vi "Execute FTE.vi"(7 "FTE":i64, 8 "error in (no error)":errorcluster, 11 "CIFCorePlugin in":refnum<class "CIFCorePlugin.lvclass">) -> (0 "error out":errorcluster, 3 "CIFCorePlugin out":refnum<class "CIFCorePlugin.lvclass">)   [LabVIEW 2021, in "CIFCorePlugin.lvclass"]
uses:
  CIFCorePlugin.lvclass
  CIFCorePlugin.lvclass/CIFCorePlugin.ctl
  <vilib>/CIF Foundation/CIF Utilities/Time/Typedef/Future Time Event Limits.ctl
  <vilib>/CIF Foundation/CIF Utilities/Time/SubVIs/Add Error.vi
  <vilib>/CIF Foundation/CIF Utilities/Time/System Time/Get System Time.vi
  <vilib>/CIF Foundation/CIF Utilities/Errors/Append Error Location.vi
  <vilib>/CIF Foundation/CIF Utilities/Time/Time_CIF_U.lvlib
  Typedef/Energized States.ctl
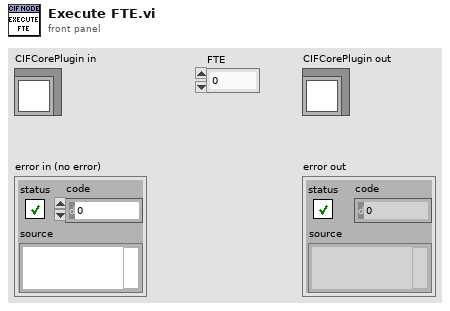
[diagram p1: front panel]
types:
  T1 = typedef "CIFCorePlugin.lvclass/Energized States.ctl" = enum16{"Listen", "Prepare", "Execute", "Housekeep", "Cleanup", "Destroy"}
  T2 = typedef "Time_CIF_U.lvlib/Future Time Event Limits.ctl" = cluster{"Maximum":i64, "Minimum":i64}
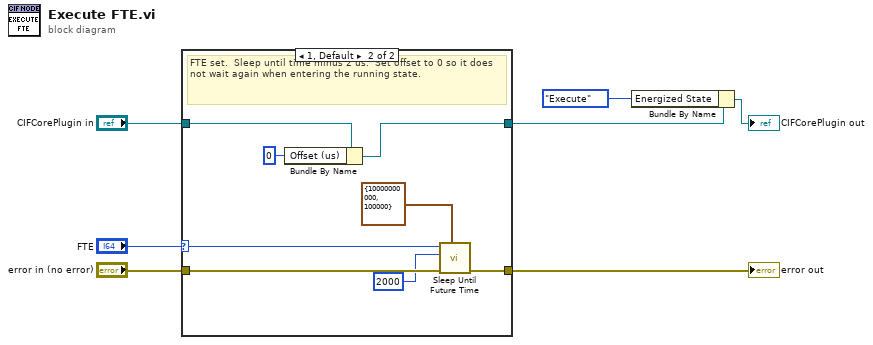
[diagram p0: block diagram]
diagram:
  n1 = case shown="1, Default" "FTE" {
    selector: "FTE" -> [_ w17]
    tunnel: [w9 w11] -> w2
    tunnel: "CIFCorePlugin in" -> [w9 w13]
    tunnel: "error in (no error)" -> [w8 w16]
    tunnel: [w8 w15] -> w4
    frame 0 {
    }
    frame 1, Default {
      # "FTE set.  Sleep until time minus 2 us.  Set offset to 0 so it does not wait again when entering the running state."
      n2 = Bundle By Name(cluster=w13, "Offset (us)"=0 ("Common Plugin Configuration.Common.Offset (us)")) -> (w11:refnum<class "CIFCorePlugin.lvclass">)
      n3 = call <vilib>:"Sleep Until Future Time.vi"("FTE Limits (ns)"=T2 {"Maximum"=10000000000, "Minimum"=100000}, "error in (no error)"=w16, "Wake Offset"=i64 2000, "Wake Time (ns)"=w17) -> ("error out"=w15:errorcluster)  [unwired: 5 in, 2 out]
    }
  }
  "error out" <- w4
  n4 = Bundle By Name(cluster=w2, "Energized State"=Energized_States."Execute") -> (→"CIFCorePlugin out":refnum<class "CIFCorePlugin.lvclass">)
